vi "PSD Scale Test.vi"() -> ()   [LabVIEW 2020]
uses:
  <vilib>/Analysis/2dsp.llb/Real FFT.vi
  <vilib>/Analysis/5stat.llb/RMS (DBL).vi
  <vilib>/addons/Time Series Analysis/Correlation and Spectral Analysis.llb/TSA Welch (Array).vi
  epl-vi-lib/Utility VIs/Conversion VIs/Create Waveform Cluster (1D).vi
  <vilib>/addons/_Advanced Signal Processing/NI_AdvSigProcTSA.lvlib
  <vilib>/Analysis/NI_AALBase.lvlib
  <vilib>/Analysis/NI_AALPro.lvlib
panel:
  out "sum 2":dbl
  out "sum":dbl
  out "rms value":dbl format="%0.2f"
  out "Waveform Graph":cluster{dbl, "dx":dbl, "Y":dbl[]}(graph)
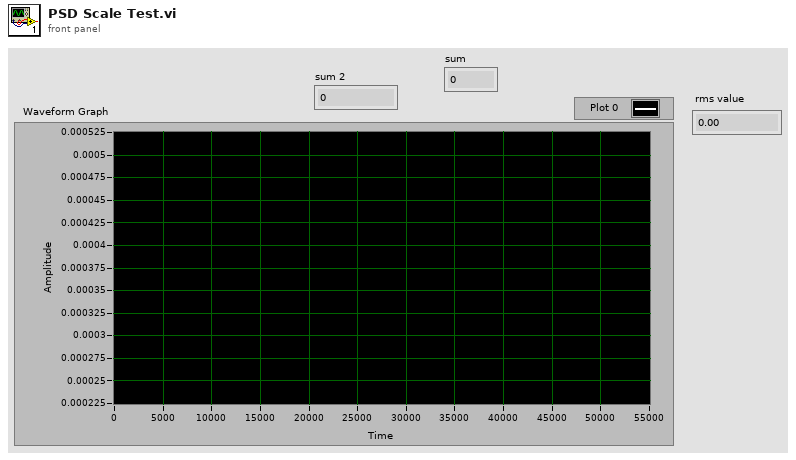
[diagram p1: front panel]
types:
  T1 = cluster{"window":u16, "length":i32, "overlap (%)":dbl}
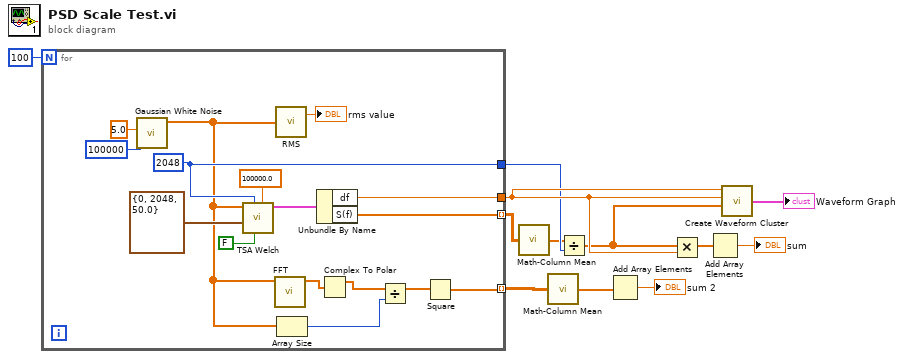
[diagram p0: block diagram]
diagram:
  n1 = for {
    N: 100 -> [_]
    tunnel: [w24] -> w7
    tunnel: [w20] -> w10 mode=indexing
    tunnel: [w19] -> w6
    tunnel: [w13] -> w3 mode=indexing
    w19 = 2048 ("length")
    n2 = call <vilib>:"Gaussian White Noise.vi"("standard deviation"=5.0, "samples"=100000) -> ("Gaussian noise pattern"=w15:dbl[])  [unwired: 8 in, 1 out]
    n3 = call-poly <vilib>:"TSA Welch.vi"("sampling rate"=100000.0, "dB on? (T)"=FALSE, "frequency bins"=w19, "window info"=T1 {"window"=0, "length"=2048, "overlap (%)"=50.0}, "Xt"=w15) -> ("PSD"=w25:cluster{"f0":dbl, "df":dbl, "S(f)":dbl[]})  [unwired: 5 in, 1 out]
    n4 = call-poly <vilib>:"FFT.vi"("X"=w15) -> ("FFT {X}"=w18:cdb[])  [unwired: 9 in, 1 out]
    n5 = call-poly <vilib>:"RMS.vi"("X"=w15) -> ("rms value"=→"rms value":dbl)  [unwired: 1 out]
    n6 = Array Size(array=w15) -> (size(s)=w14:i32)
    n7 = Unbundle By Name(w25) -> ("df"=w24:dbl, "S(f)"=w20:dbl[])
    n8 = Complex To Polar(r * e^(i*theta)=w18) -> (r=w17:dbl[])  [unwired: 1 out]
    n9 = Divide(x=w17, y=w14) -> (x/y=w16:dbl[])
    n10 = Square(x=w16) -> (x^2=w13:dbl[])
  }
  n11 = call "Math-Column Mean.vi"("2D Array"=w10) -> ("Column means"=w5:dbl[])
  n12 = call "Math-Column Mean.vi"("2D Array"=w3) -> ("Column means"=w1:dbl[])
  n13 = Divide(x=w5, y=w6) -> (x/y=w4:dbl[])
  n14 = Add Array Elements(numeric array=w1) -> (sum=→"sum 2":dbl)
  n15 = Multiply(x=w4, y=w7) -> (x*y=w9:dbl[])
  n16 = Add Array Elements(numeric array=w9) -> (sum=→"sum":dbl)
  n17 = call-poly "Create Waveform Cluster.vi"("dx"=w7, "Y"=w4, "offset"=w7) -> ("waveform cluster"=→"Waveform Graph":cluster{dbl, "dx":dbl, "Y":dbl[]})  [unwired: 2 in]
